vi "set_number_of_frames.vi"(8 "error in (no error)":errorcluster, 10 "number of frames":i32, 11 "ScanModeMG090624Camera in":refnum<class "ScanModeMG090624Camera.lvclass">=refnum) -> (0 "error out":errorcluster, 3 "ScanModeMG090624Camera out":refnum<class "ScanModeMG090624Camera.lvclass">)   [LabVIEW 2010]
uses:
  ScanModeMG090624Camera.lvclass
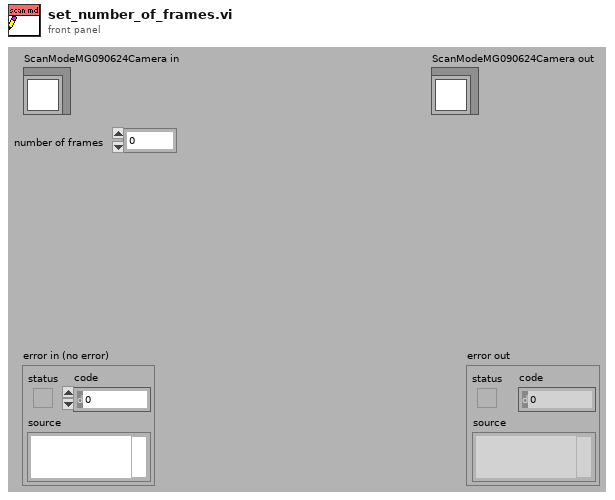
[diagram p1: front panel]
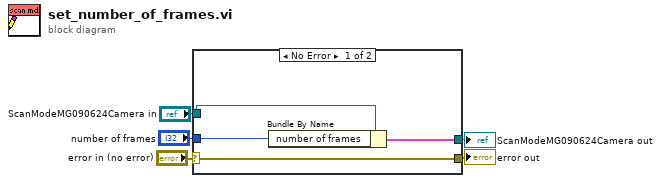
[diagram p0: block diagram]
diagram:
  n1 = case shown="No Error" "error in (no error)" {
    selector: "error in (no error)" -> [w9 w10]
    tunnel: [w9 w10] -> w4
    tunnel: [w7 w11] -> w2
    tunnel: "ScanModeMG090624Camera in" -> [w8 w11]
    tunnel: "number of frames" -> [w6 _]
    frame No Error {
      n2 = Bundle By Name(cluster=w8, "number of frames"=w6) -> (w7:cluster{})
    }
    frame Error {
    }
  }
  "error out" <- w4
  "ScanModeMG090624Camera out" <- w2
